vi "scan1line.vi"(6 "dwell_time_ms":dbl=0.1 format="%#_6p", 8 "error in (no error)":errorcluster, 9 "q_pixels":i32=100, 10 "y_end":dbl=10.0 min=-10.0 max=10.0 format="%.3f", 11 "y_start":dbl=-10.0 min=-10.0 max=10.0 format="%.3f") -> (0 "error out":errorcluster, 3 "histogram plot":dbl[](graph)=[0.0, 0.0, 3000.0, 4000.0, 0.0, 0.0, 1000.0, 0.0, 0.0, 3000.0, 0.0, 1000.0, 0.0, 2000.0, 0.0, 0.0, 1000.0, 0.0, 2000.0, 1000.0, 4000.0, 0.0, 0.0, 0.0, 0.0, 0.0, 8000.0, 0.0, 0.0, 0.0, 1000.0, 0.0, 5000.0, 0.0, 0.0, 0.0, 0.0, 2000.0, 5000.0, 0.0, 0.0, 0.0, 0.0, 3000.0, 3000.0, 0.0, 0.0, 0.0, 1000.0, 2000.0, 1000.0, 0.0, 0.0, 1000.0, 0.0, 1000.0, 2000.0, 0.0, 2000.0, 0.0, 0.0, 0.0, 2000.0, 0.0, 0.0, 0.0, 0.0, 3000.0, 1000.0, 0.0, 0.0, 0.0, 1000.0, 3000.0, 3000.0, 0.0, 0.0, 2000.0, 0.0, 6000.0, 0.0, 1000.0, 1000.0, 0.0, 2000.0, 4000.0, 0.0, 0.0, 0.0, 0.0, 0.0, 0.0, 0.0, 1000.0, 0.0, 0.0, 2000.0, 2000.0, 0.0, 0.0])   [LabVIEW 2018]
uses:
  GLOBAL_VAR.vi
panel:
  in  "filter":bool=TRUE
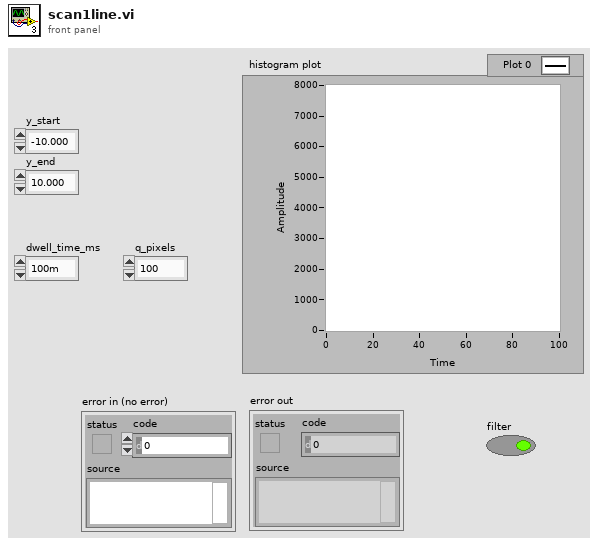
[diagram p1: front panel]
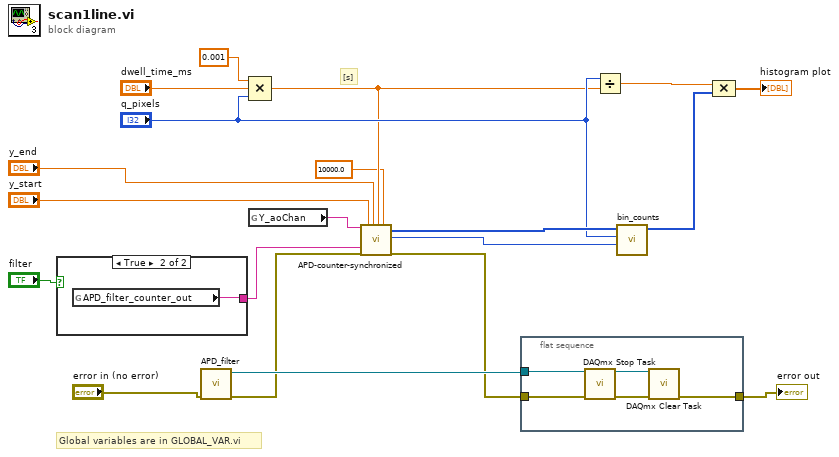
[diagram p0: block diagram]
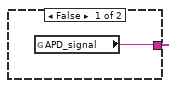
[diagram p2: hidden frame]
diagram:
  # "[s]"
  # "Global variables are in GLOBAL_VAR.vi"
  n1 = case shown="True" "filter" {
    tunnel: [w21 w22] -> w10
    frame False {
      n2 = global read "GLOBAL_VAR.vi" "APD_signal"() -> (w21:tag)
    }
    frame True {
      n3 = global read "GLOBAL_VAR.vi" "APD_filter_counter_out"() -> (w22:tag)
    }
  }
  n4 = call "APD_filter.vi"("error in"="error in (no error)") -> ("error out"=w11:errorcluster, "filtered APD"=w19:refnum<k21>)  [unwired: 5 in]
  n5 = Compound Arithmetic op=MULTIPLY(0.001 ("value"), "dwell_time_ms", "q_pixels") -> (w5:dbl)
  n6 = global read "GLOBAL_VAR.vi" "Y_aoChan"() -> (w15:tag)
  n7 = call "APD-counter-synchronized.vi"("ao_to_write"=w15, "APD_signal"=w10, "error in (no error)"=w11, "y_start_um"="y_start", "y_end_um"="y_end", "Duration_s"=w5, "DAQ sampling rate"=10000.0) -> ("time tags"=w14:u32[], "clock cycles"=w13:i32, "error out"=w12:errorcluster)  [unwired: 9 in, 1 out]
  n8 = flat-sequence {
    tunnel: w19 -> [w25]
    tunnel: w12 -> [w24]
    tunnel: [w23] -> w18
    frame #0 {
      n9 = call <vilib>:"DAQmx Stop Task.vi"("task/channels in"=w25, "error in"=w24) -> ("task out"=w27:refnum<k21>, "error out"=w26:errorcluster)  [unwired: 12 in]
      n10 = call <vilib>:"DAQmx Clear Task.vi"("task in"=w27, "error in"=w26) -> ("error out"=w23:errorcluster)  [unwired: 13 in]
    }
  }
  n11 = Divide(x="q_pixels", y=w5) -> (x/y=w4:dbl)
  n12 = call "bin_counts.vi"("#clock cycles"=w13, "#bins"="q_pixels", "counter timetag list"=w14) -> ("histogram"=w3:i32[])  [unwired: 4 in, 3 out]
  n13 = Compound Arithmetic op=MULTIPLY(w4, w3) -> (→"histogram plot":dbl[])
  "error out" <- w18
